vi "make_request.vi"(5 "Content-Type":string, 7 "Method":string="get", 8 "Error in":errorcluster, 9 "payload":string, 10 "path":string="/api/documents", 11 "Device In":T2) -> (0 "error out":errorcluster, 2 "Comm":T1)   [LabVIEW 2019]
uses:
  <userlib>/IoT Devices/_subVIs/HTTPComm.ctl
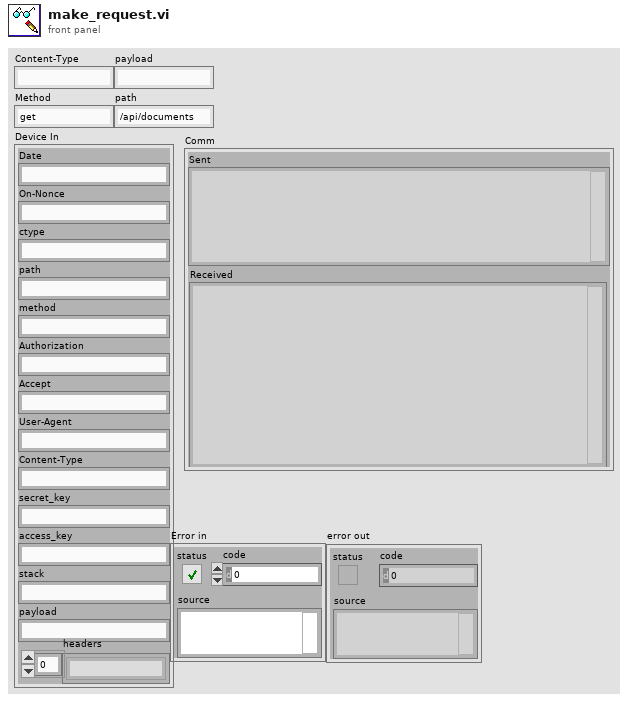
[diagram p1: front panel]
types:
  T1 = typedef "HTTPComm.ctl" = cluster{"url":string, "sent headers":string, "sent body":string, "headers":string, "body":string, "Sent":string, "Received":string}
  T2 = cluster{"Date":string, "On-Nonce":string, "ctype":string, "path":string, "method":string, "Authorization":string, "Accept":string, "User-Agent":string, "Content-Type":string, "secret_key":string, "access_key":string, "stack":string, "payload":string, "headers":string[]}
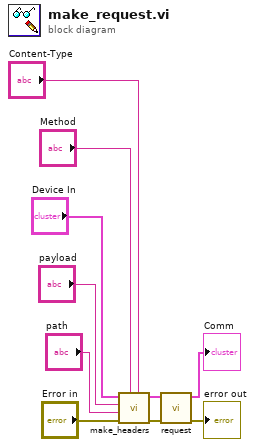
[diagram p0: block diagram]
diagram:
  n1 = call "make_headers.vi"("Content-Type"="Content-Type", "Method"="Method", "Error in"="Error in", "path"="path", "payload"="payload", "Device In"="Device In") -> ("Error Out"=w9:errorcluster, "Device Out"=w10:T2)  [unwired: 4 in]
  n2 = call "request.vi"("Device In"=w10, "error in"=w9) -> ("Comm"=→"Comm":T1, "error out"=→"error out":errorcluster)  [unwired: 7 in]
